vi "CheckWinRow(SubVI).vi"(11 "Array":string[][](array[string])) -> (3 "x .or. y? 2":bool)   [LabVIEW 2020]
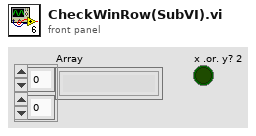
[diagram p1: front panel]
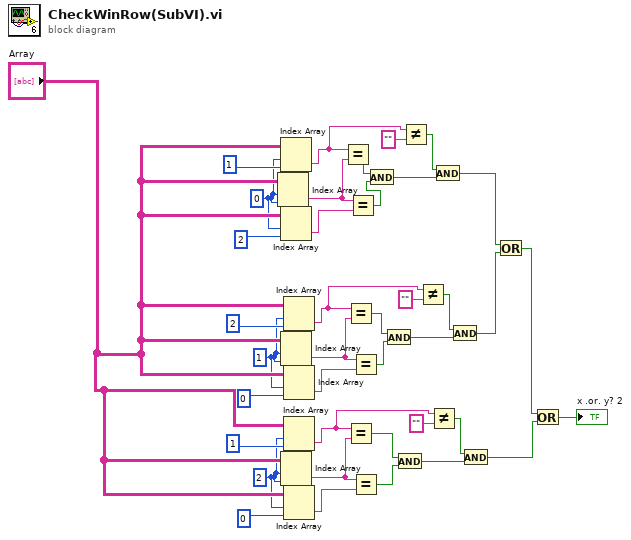
[diagram p0: block diagram]
diagram:
  w11 = 2
  w6 = 1
  w1 = 0
  n1 = Index Array(array="Array", index (row)=w1, index (col)=w1) -> (element=w4:string)
  n2 = Index Array(array="Array", index (row)=w1, index (col)=1) -> (element=w31:string)
  n3 = Index Array(array="Array", index (row)=w1, index (col)=2) -> (element=w5:string)
  n4 = Index Array(array="Array", index (row)=w6, index (col)=w6) -> (element=w9:string)
  n5 = Index Array(array="Array", index (row)=w11, index (col)=w11) -> (element=w14:string)
  n6 = Index Array(array="Array", index (row)=w6, index (col)=2) -> (element=w27:string)
  n7 = Index Array(array="Array", index (row)=w6, index (col)=0) -> (element=w10:string)
  n8 = Index Array(array="Array", index (row)=w11, index (col)=1) -> (element=w19:string)
  n9 = Index Array(array="Array", index (row)=w11, index (col)=0) -> (element=w15:string)
  n10 = Equal?(x=w31, y=w4) -> (x = y?=w32:bool)
  n11 = Equal?(x=w27, y=w9) -> (x = y?=w25:bool)
  n12 = Equal?(x=w19, y=w14) -> (x = y?=w16:bool)
  n13 = Equal?(x=w4, y=w5) -> (x = y?=w33:bool)
  n14 = Equal?(x=w9, y=w10) -> (x = y?=w26:bool)
  n15 = Equal?(x=w14, y=w15) -> (x = y?=w17:bool)
  n16 = And(x=w32, y=w33) -> (x .and. y?=w29:bool)
  n17 = And(x=w25, y=w26) -> (x .and. y?=w23:bool)
  n18 = And(x=w16, y=w17) -> (x .and. y?=w20:bool)
  n19 = Not Equal?(x=w31, y="") -> (x != y?=w30:bool)
  n20 = Not Equal?(x=w27, y="") -> (x != y?=w24:bool)
  n21 = Not Equal?(x=w19, y="") -> (x != y?=w21:bool)
  n22 = And(x=w30, y=w29) -> (x .and. y?=w34:bool)
  n23 = And(x=w24, y=w23) -> (x .and. y?=w35:bool)
  n24 = And(x=w21, y=w20) -> (x .and. y?=w37:bool)
  n25 = Or(x=w34, y=w35) -> (x .or. y?=w36:bool)
  n26 = Or(x=w36, y=w37) -> (x .or. y?=→"x .or. y? 2":bool)
